vi "Kalman loop (SubVI).vi"(3 "DT":dbl, 4 "Array":dbl[][](array[numeric]), 5 "Constants":T1) -> (0 "Acc":dbl[](array[numeric]), 1 "Gyro":dbl[](array[numeric]), 2 "Angles":dbl[](array[numeric]))   [LabVIEW 2013]
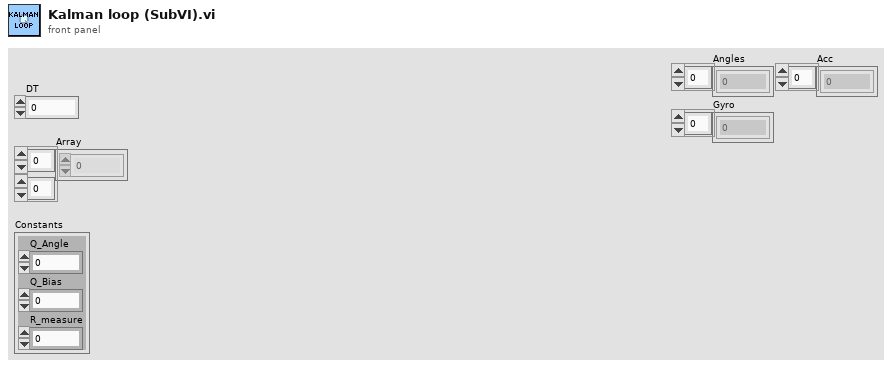
[diagram p1: front panel]
types:
  T1 = cluster{"Q_Angle":dbl, "Q_Bias":dbl, "R_measure":dbl}
  T2 = cluster{"Array[0]":dbl, "Array[1]":dbl, "Array[2]":dbl, "Array[3]":dbl, "Array[4]":dbl, "Array[5]":dbl, "Array[6]":dbl, "Array[7]":dbl, "Array[8]":dbl}
  T3 = cluster{"Array[1]":dbl, "Array[0]":dbl, "DT":dbl}
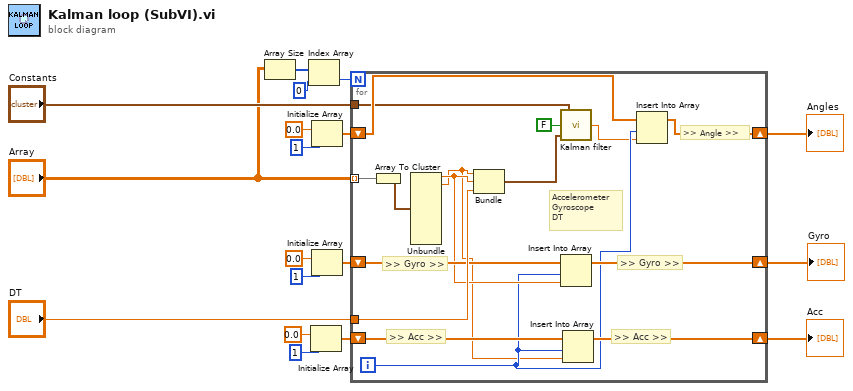
[diagram p0: block diagram]
diagram:
  n1 = Array Size(array="Array") -> (size(s)=w5:i32[])
  n2 = Index Array(array=w5, index=0) -> (element=w9:i32)
  n3 = Initialize Array(0.0 ("element"), 1 ("dimension size")) -> (w14:dbl[])
  n4 = Initialize Array(0.0 ("element"), 1 ("dimension size")) -> (w17:dbl[])
  n5 = Initialize Array(0.0 ("element"), 1 ("dimension size")) -> (w11:dbl[])
  n6 = for {
    N: w9 -> [_]
    tunnel: "Array" -> [w33] mode=indexing
    tunnel: "DT" -> [w31]
    shift-right: [w28] -> w2
    shift-left: w11 -> [w29]
    shift-right: [w25] -> w1
    shift-left: w14 -> [w26]
    shift-right: [w23] -> w3
    shift-left: w17 -> [w24]
    tunnel: "Constants" -> [w19]
    i -> [w22]
    # ">> Angle >>"
    # ">> Acc >>"
    # ">> Acc >>"
    # ">> Gyro >>"
    # ">> Gyro >>"
    # "Accelerometer\nGyroscope\nDT"
    n7 = Array To Cluster(array=w33) -> (cluster=w32:T2)
    n8 = Unbundle(w32) -> ("Array[0]"=w27:dbl, "Array[1]"=w21:dbl)  [unwired: 7 out]
    n9 = Bundle("Array[1]"=w21, "Array[0]"=w27, "DT"=w31) -> (w30:T3)  [unwired: 1 in]
    n10 = call "Kalman filter.vi"("New data"=w30, "Reset"=FALSE, "Constants"=w19) -> ("Angle out"=w20:dbl)
    n11 = Insert Into Array(array=w29, index=w22, new element=w27) -> (w28:dbl[])
    n12 = Insert Into Array(array=w26, index=w22, new element=w21) -> (w25:dbl[])
    n13 = Insert Into Array(array=w24, index=w22, new element=w20) -> (w23:dbl[])
  }
  "Angles" <- w3
  "Gyro" <- w2
  "Acc" <- w1
